vi "Get All Fitting Parameters from folders.vi"() -> ()   [LabVIEW 2014]
uses:
  <vilib>/Analysis/baseanly.llb/Mean (DBL).vi
  <vilib>/Utility/file.llb/Read From Spreadsheet File (DBL).vi
  <vilib>/Utility/file.llb/Write To Spreadsheet File (DBL).vi
  <vilib>/Analysis/NI_AALBase.lvlib
panel:
  out "concatenated string":string
  out "N":i32
  out "transposed array":dbl[][](array[numeric])
  out "All Folders":path[](array[path])
  in  "Save?":bool
  out "K":dbl[](array[numeric])
  out "Lc":dbl[](array[numeric])
  out "Lp":dbl[](array[numeric])
  in  "Folder Path":path
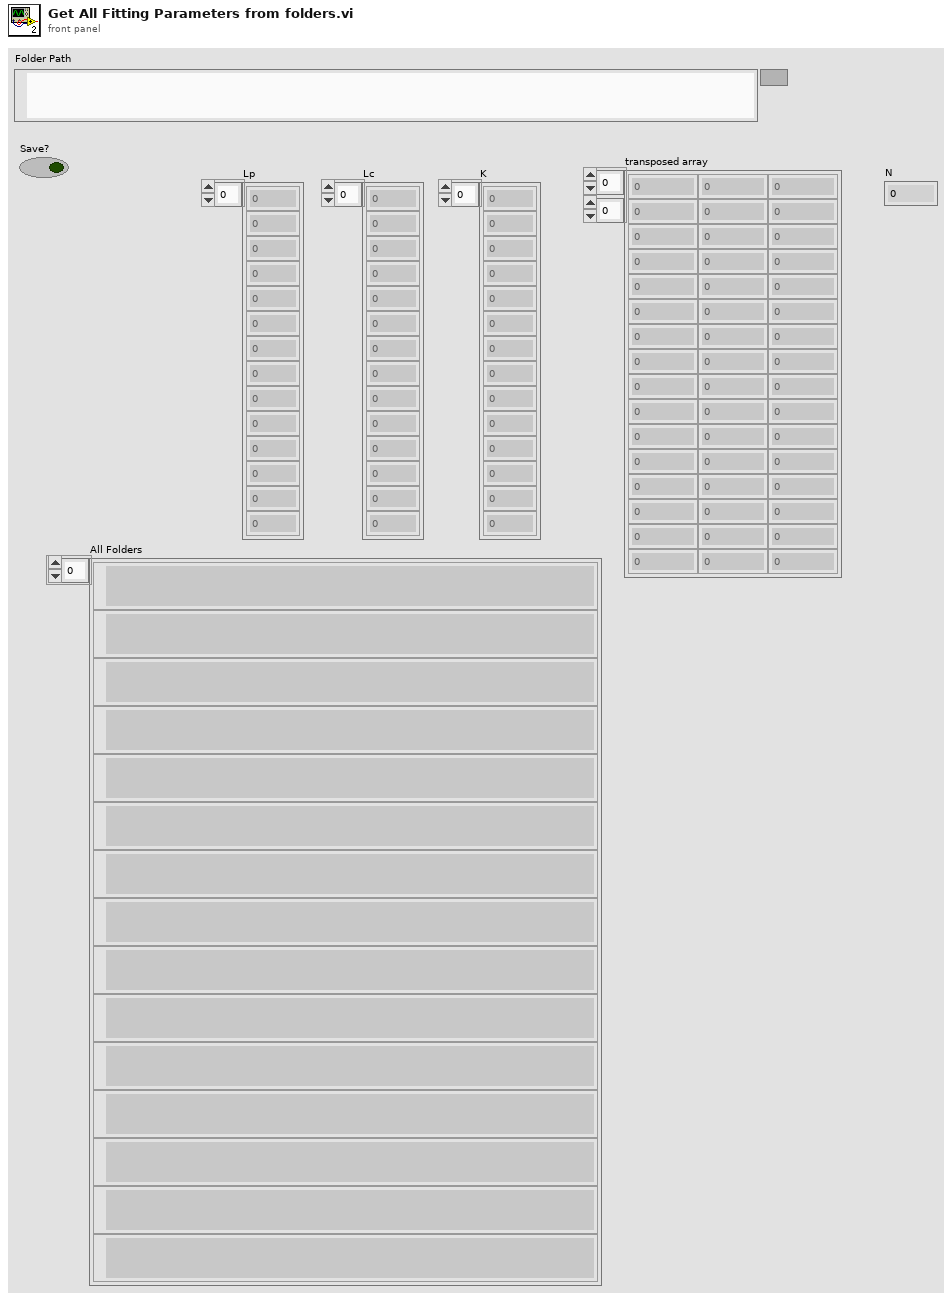
[diagram p1: front panel]
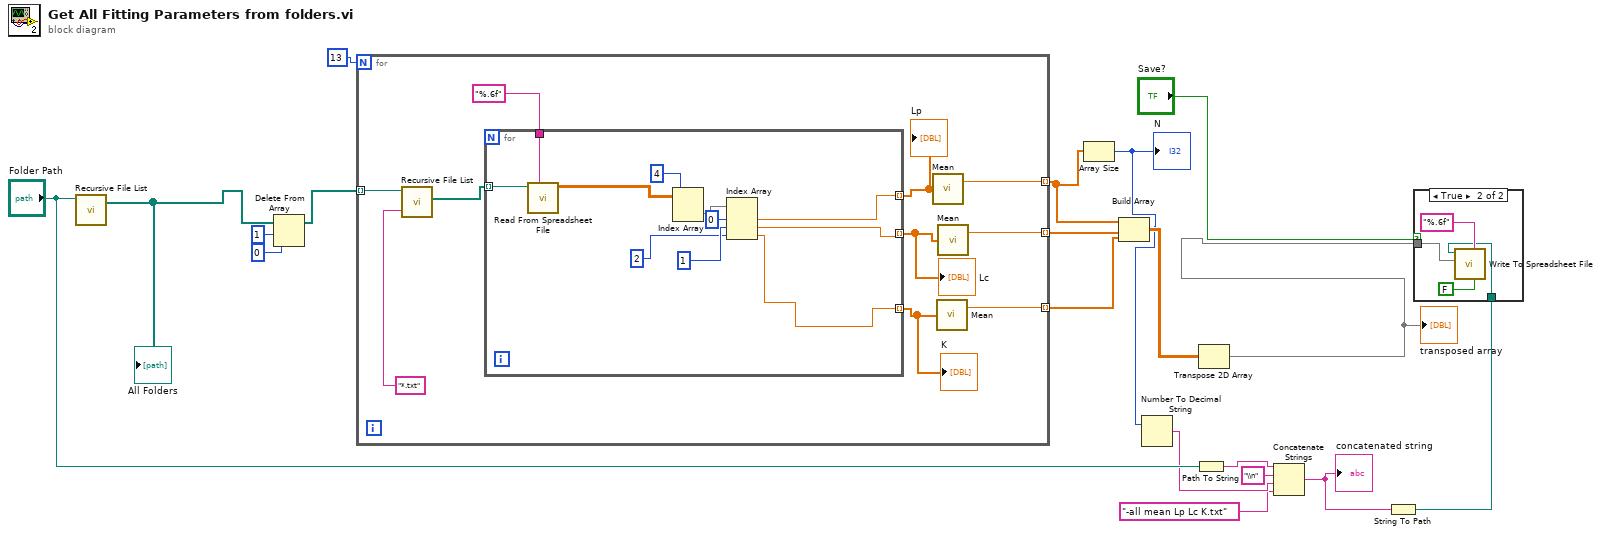
[diagram p0: block diagram]
diagram:
  n1 = call <vilib>:"Recursive File List.vi"("Folder Path"="Folder Path") -> ("All Folders"=w16:path[])  [unwired: 6 in, 4 out]
  "All Folders" <- w16
  n2 = Delete From Array(array=w16, length=1, index=0) -> (array with subset deleted=w13:path[])  [unwired: 1 out]
  n3 = for {
    N: 13 -> [_]
    tunnel: w13 -> [w29] mode=indexing
    tunnel: [w25] -> w9 mode=indexing
    tunnel: [w24] -> w19 mode=indexing
    tunnel: [w23] -> w18 mode=indexing
    n4 = call <vilib>:"Recursive File List.vi"("pattern"="*.txt", "Folder Path"=w29) -> ("All Files in Dir"=w26:path[])  [unwired: 5 in, 4 out]
    n5 = for {
      tunnel: "%.6f" ("format (%.3f)") -> [w40]
      tunnel: w26 -> [w35] mode=indexing
      tunnel: [w32] -> w22 mode=indexing
      tunnel: [w31] -> w21 mode=indexing
      tunnel: [w30] -> w20 mode=indexing
      n6 = call-poly <vilib>:"Read From Spreadsheet File.vi"("format (%.3f)"=w40, "file path (dialog if empty)"=w35) -> ("all rows"=w39:dbl[][])  [unwired: 5 in, 4 out]
      n7 = Index Array(array=w39, index (col)=4 ("disabled index (col)")) -> (element=w37:dbl[])  [unwired: 1 in]
      n8 = Index Array(array=w37, index #1=0 ("index"), index #2=1 ("index"), index #3=2 ("index")) -> (element #1=w32:dbl, element #2=w31:dbl, element #3=w30:dbl)
    }
    "Lp" <- w22
    "Lc" <- w21
    "K" <- w20
    n9 = call-poly <vilib>:"Mean.vi"("X"=w22) -> ("mean"=w25:dbl)  [unwired: 1 out]
    n10 = call-poly <vilib>:"Mean.vi"("X"=w20) -> ("mean"=w23:dbl)  [unwired: 1 out]
    n11 = call-poly <vilib>:"Mean.vi"("X"=w21) -> ("mean"=w24:dbl)  [unwired: 1 out]
  }
  n12 = Array Size(array=w9) -> (size(s)=w5:i32)
  "N" <- w5
  n13 = Build Array(w9, w19, w18) -> (w11:dbl[][])
  n14 = Number To Decimal String(number=w5) -> (decimal integer string=w4:string)  [unwired: 1 in]
  n15 = Path To String(path="Folder Path") -> (string=w6:string)
  n16 = Transpose 2D Array(2D array=w11) -> (transposed array=w10:dbl[][])
  "transposed array" <- w10
  n17 = Concatenate Strings(w6, "\\n" ("string"), w4, "-all mean Lp Lc K.txt" ("string")) -> (w2:string)
  "concatenated string" <- w2
  n18 = String To Path(string=w2) -> (path=w1:path)
  n19 = case shown="True" "Save?" {
    tunnel: w10 -> [_ w44]
    tunnel: w1 -> [_ w41]
    frame False {
    }
    frame True {
      n20 = call-poly <vilib>:"Write To Spreadsheet File.vi"("transpose? (no:F)"=FALSE, "format (%.3f)"="%.6f", "2D data"=w44, "file path (dialog if empty)"=w41) -> ()  [unwired: 4 in, 1 out]
    }
  }
